vi "Find Center Setup.vi"(6 "XYZTheta":dbl[](array[numeric]), 8 "Assembly Type":string, 9 "Position":i32, 10 "Tray Number":dbl format="%#_13g", 11 "Carrier Tray":T1) -> (3 "Assembly Tray Out":T1)   [LabVIEW 2021, in "Assembly Tray.lvclass"]
uses:
  Assembly Tray.lvclass
  Find Tray.ctl
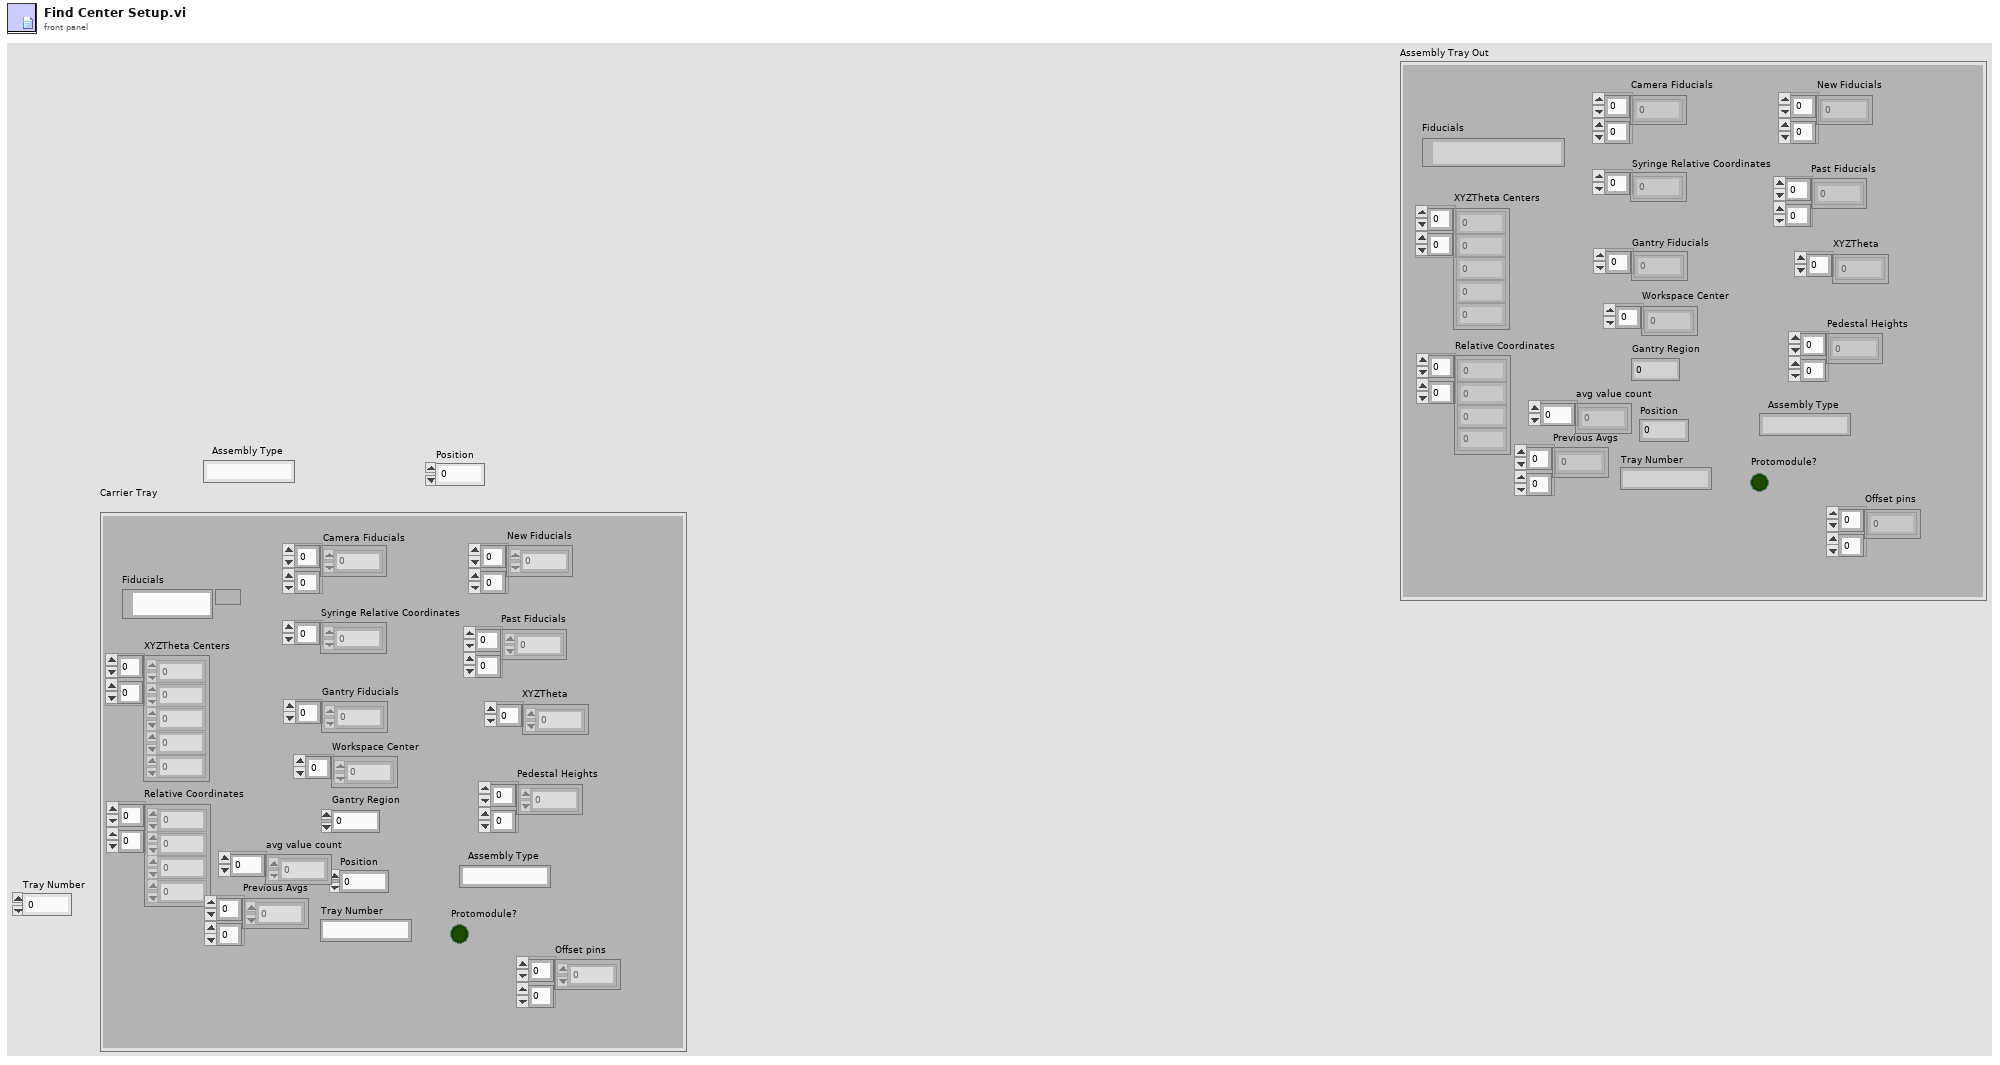
[diagram p1: front panel]
types:
  T1 = typedef "Assembly Tray.lvclass/Find Tray.ctl" = cluster{"Gantry Fiducials":dbl[], "Relative Coordinates":dbl[][], "Camera Fiducials":dbl[][], "XYZTheta Centers":dbl[][], "Workspace Center":dbl[], "Syringe Relative Coordinates":dbl[], "Gantry Region":dbl, "Fiducials":path, "New Fiducials":dbl[][], "Past Fiducials":dbl[][], "XYZTheta":dbl[], "Pedestal Heights":dbl[][], "Assembly Type":string, "Tray Number":string, "Position":i32, "Protomodule?":bool, "avg value count":dbl[], "Previous Avgs":dbl[][], "Offset pins":dbl[][]}
  T2 = typedef "File Paths.ctl" = cluster{"Glue Pattern Folder":path, "Carrier Tray Folder":path, "Pick Up Tool Fixture Folder":path, "Components Folder":path, "Bellows Tool Offset.txt":path, "Pick Up Tool Offset.txt":path, "Dispense Tip Offset.txt":path, "Log Files":path, "Gantry Assembly Map.txt":path, "Syringe and offset map.txt":path, "Controllers Folder":path, "Local dbase config":path}
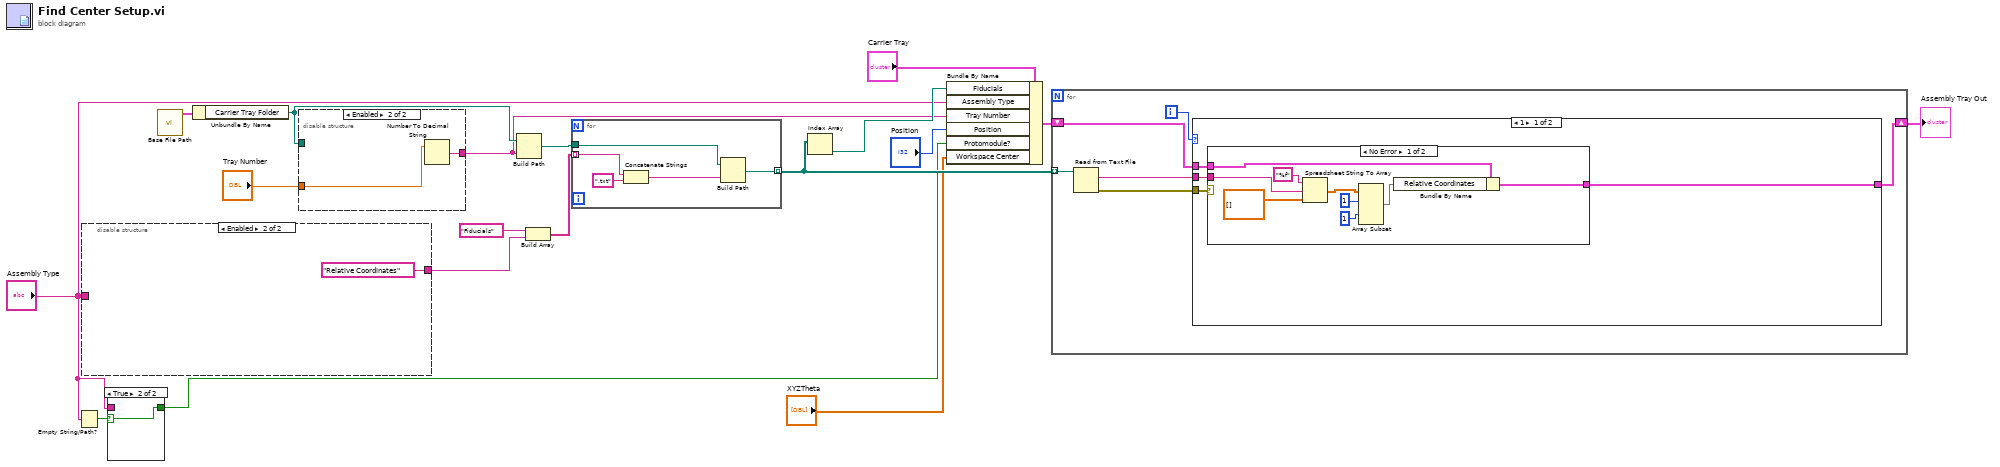
[diagram p0: block diagram]
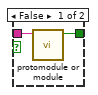
[diagram p2: hidden frame]
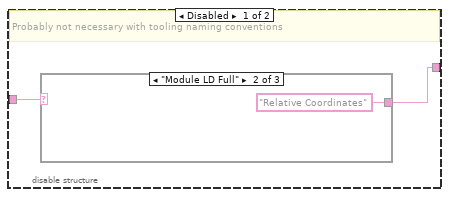
[diagram p3: hidden frame]
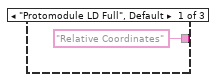
[diagram p4: hidden frame]
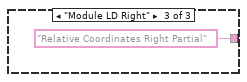
[diagram p5: hidden frame]
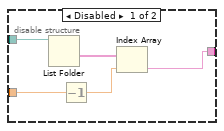
[diagram p6: hidden frame]
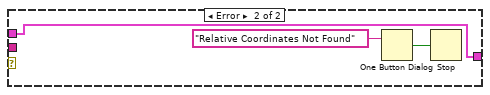
[diagram p7: hidden frame]
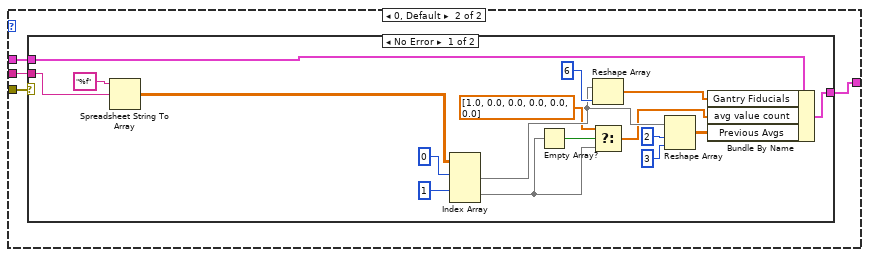
[diagram p8: hidden frame]
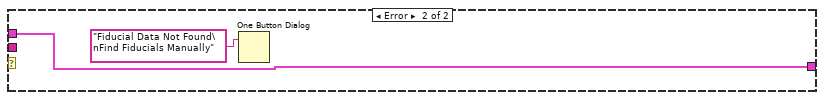
[diagram p9: hidden frame]
diagram:
  n1 = Empty String/Path?(string/path="Assembly Type") -> (empty?=w3:bool)
  n2 = disable-structure shown="Enabled" {
    disable-tunnel: [w20 "Relative Coordinates" ("format string")] -> w12
    disable-tunnel: "Assembly Type" -> [w19 _]
    frame Disabled {
      # "Probably not necessary with tooling naming conventions"
      n3 = case shown="\"Module LD Full\"" w19 {
        tunnel: ["Relative Coordinates" ("format string") "Relative Coordinates" ("format string") "Relative Coordinates Right Partial" ("format string")] -> w20
        frame "Protomodule LD Full", Default {
        }
        frame "Module LD Full" {
        }
        frame "Module LD Right" {
        }
      }
    }
    frame Enabled {
    }
  }
  n4 = case shown="True" w3 {
    selector: w3 -> [_ w27]
    tunnel: "Assembly Type" -> [w26 _]
    tunnel: [w25 w27] -> w1
    frame False {
      n5 = call "protomodule or module.vi"("assembly type"=w26) -> ("protomodule? (T)"=w25:bool)  [unwired: 10 in]
    }
    frame True {
    }
  }
  n6 = call "Base File Path.vi"() -> ("Paths Out"=w15:T2)  [unwired: 11 in]
  n7 = Unbundle By Name(w15) -> ("Carrier Tray Folder"=w9:path)
  n8 = disable-structure shown="Enabled" {
    disable-tunnel: [w31 w33] -> w6
    disable-tunnel: "Tray Number" -> [w29 w34]
    disable-tunnel: w9 -> [w28 _]
    frame Disabled {
      n9 = List Folder(path=w28) -> (folder names=w32:string[])  [unwired: 3 in, 3 out]
      n10 = Decrement(x=w29) -> (x-1=w30:dbl)
      n11 = Index Array "Index Array"(array=w32, index=w30) -> (element=w31:string)
    }
    frame Enabled {
      n12 = Number To Decimal String(number=w34) -> (decimal integer string=w33:string)  [unwired: 1 in]
    }
  }
  n13 = Build Path(base path=w9, name or relative path=w6) -> (appended path=w10:path)
  n14 = Build Array("Fiducials" ("format string"), w12) -> (w16:string[])
  n15 = for {
    tunnel: w16 -> [w38] mode=indexing
    tunnel: w10 -> [w39]
    tunnel: [w35] -> w11 mode=indexing
    n16 = Concatenate Strings "Concatenate Strings"(w38, ".txt" ("string")) -> (w36:string)
    n17 = Build Path(base path=w39, name or relative path=w36) -> (appended path=w35:path)
  }
  n18 = Index Array "Index Array"(array=w11) -> (element=w17:path)  [unwired: 1 in]
  n19 = Bundle By Name "Bundle By Name"(cluster="Carrier Tray", "Fiducials"=w17, "Assembly Type"="Assembly Type", "Tray Number"=w6, "Position"="Position", "Protomodule?"=w1, "Workspace Center"="XYZTheta") -> (w18:T1)
  n20 = for {
    tunnel: w11 -> [w44] mode=indexing
    shift-right: [w40] -> w14
    shift-left: w18 -> [w41]
    i -> [w42]
    n21 = Read from Text File(file (use dialog)=w44) -> (text=w45:string, error out=w43:errorcluster)  [unwired: 3 in, 2 out]
    n22 = case shown="1" w42 {
      tunnel: w45 -> [w48 w65]
      tunnel: w43 -> [w49 w64]
      tunnel: w41 -> [w47 w63]
      tunnel: [w46 w62] -> w40
      frame 1 {
        n23 = case shown="No Error" w49 {
          tunnel: w48 -> [w56 _]
          tunnel: [w54 w59] -> w46
          tunnel: w47 -> [w55 w59]
          frame No Error {
            n24 = Spreadsheet String To Array(format string="%f", spreadsheet string=w56, array type (2D Dbl)=dbl[][] []) -> (array=w53:dbl[][])  [unwired: 1 in]
            n25 = Array Subset(array=w53, index (row)=1 ("length"), index (col)=1 ("index (row)")) -> (w52:dbl[][])  [unwired: 2 in]
            n26 = Bundle By Name(cluster=w55, "Relative Coordinates"=w52) -> (w54:T1)
          }
          frame Error {
            n27 = One Button Dialog(message="Relative Coordinates Not Found") -> (true=w60:bool)  [unwired: 1 in]
            n28 = Stop(stop? (T)=w60) -> ()
          }
        }
      }
      frame 0, Default {
        n29 = case shown="No Error" w64 {
          tunnel: w65 -> [w81 _]
          tunnel: w63 -> [w79 w83]
          tunnel: [w80 w83] -> w62
          frame No Error {
            n30 = Spreadsheet String To Array(format string="%f", spreadsheet string=w81) -> (array=w77:dbl[][])  [unwired: 2 in]
            n31 = Index Array "Index Array"(array=w77, index (row) #1=0 ("index (row)"), index (row) #2=1 ("index (row)")) -> (element #1=w74:dbl[], element #2=w69:dbl[])  [unwired: 2 in]
            n32 = Empty Array?(array=w69) -> (empty?=w70:bool)
            n33 = Reshape Array "Reshape Array"(w74, 6 ("dimension size")) -> (w78:dbl[])
            n34 = Select(t=dbl[] [1.0, 0.0, 0.0, 0.0, 0.0, 0.0], s=w70, f=w69) -> (s? t:f=w68:dbl[])
            n35 = Reshape Array(w74, 2 ("dimension size"), 3 ("dimension size")) -> (w71:dbl[][])
            n36 = Bundle By Name "Bundle By Name"(cluster=w79, "Gantry Fiducials"=w78, "avg value count"=w68, "Previous Avgs"=w71) -> (w80:T1)
          }
          frame Error {
            n37 = One Button Dialog(message="Fiducial Data Not Found\nFind Fiducials Manually") -> ()  [unwired: 1 in, 1 out]
          }
        }
      }
    }
  }
  "Assembly Tray Out" <- w14
